vi "McPherson Setup for new pi.vi"(0 "Old GOTO":dbl format="%.2f", 2 "Old Begin":dbl format="%.2f", 4 "Old End":dbl format="%.2f", 7 "Duration":dbl format="%.2f", 9 "New Wavelength Unit":T1, 10 "Grating Density (g/mm)":T2=enum."1200" caption="Grating Density") -> (11 "Min Scan Time":dbl format="%.2f", 12 "StepperOutput":T3, 13 "Display":T4 {"Range"."Increment" format="%.2f"; "Range"."Maximum" format="%.2f"; "Range"."Minimum" format="%.2f"}, 14 "New GOTO":dbl format="%.2f", 16 "New Begin":dbl format="%.2f", 18 "New End":dbl format="%.2f", 19 "StepperGotoZ":i32)   [LabVIEW 2019]
uses:
  Globals and TypeDefs/Type Definitions.llb/McPherson Grating Density.ctl
  Globals and TypeDefs/Type Definitions.llb/Wavelength Unit.ctt
  File and save/X-Axis Converter.llb/X-Axis Converter.vi
panel:
  out "EndStep":i32
  out "BeginStep":i32
  out "Speed Output":i16
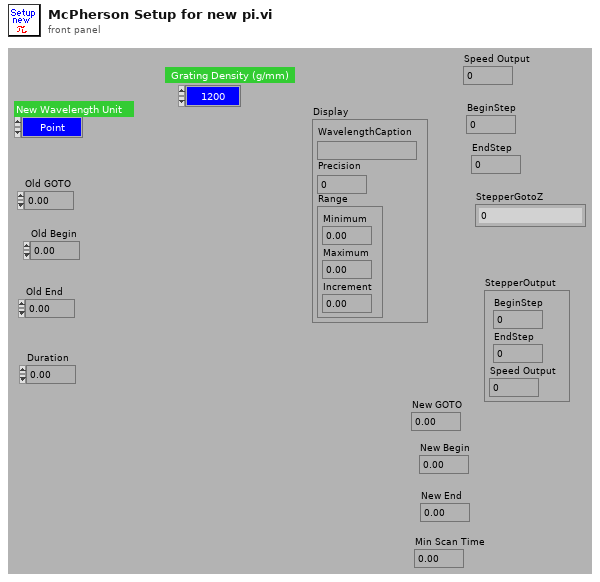
[diagram p1: front panel]
types:
  T1 = typedef "Wavelength Unit.ctt" = enum8{"Point", "nm", "eV", "meV", "cm_1"}
  T2 = typedef "McPherson Grating Density.ctl" = enum8{"150", "300", "600", "1200", "1800"}
  T3 = cluster{"BeginStep":i32, "EndStep":i32, "Speed Output":i16}
  T4 = cluster{"WavelengthCaption":string, "Precision":u8, "Range":cluster{"Minimum":dbl, "Maximum":dbl, "Increment":dbl}}
  T5 = cluster{"X-Axis Unit String":string, "Precision":i32, cluster{dbl, dbl, dbl}}
  T6 = cluster{"Stepper Position Output":i32, "Stepper Position Output":i32, i16}
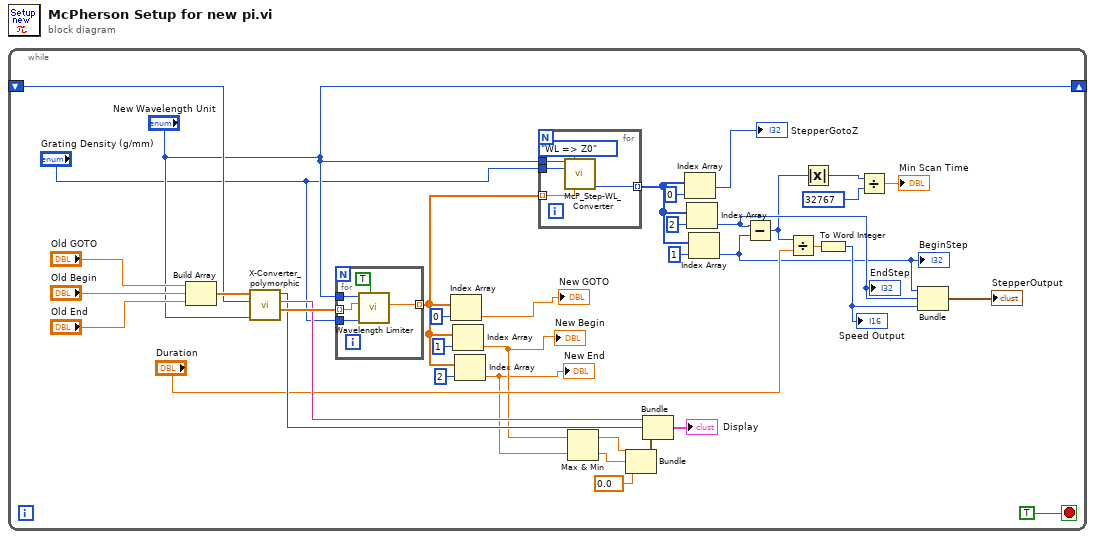
[diagram p0: block diagram]
diagram:
  n1 = while {
    shift-right: ["New Wavelength Unit"] -> _
    shift-left: _ -> [w12]
    stop <- TRUE stop-if-true
    n2 = Build Array("Old GOTO", "Old Begin", "Old End") -> (w15:dbl[])
    n3 = call-poly "X-Converter_polymorphic.vi"("X-Axis Unit"="New Wavelength Unit", "Old X-Axis Unit"=w12, "X-Axis input"=w15) -> ("X-Axis Output"=w36:dbl[], "X-Axis Unit String"=w24:string, "Precision"=w22:i32)  [unwired: 2 in, 1 out]
    n4 = for {
      tunnel: w36 -> [w48] mode=indexing
      tunnel: "New Wavelength Unit" -> [w47]
      tunnel: "Grating Density (g/mm)" -> [w46]
      tunnel: [w45] -> w32 mode=indexing
      n5 = call "Wavelength Limiter.vi"("Range Limiter(F) or WL limiter"=TRUE, "Current Grating Density"=w46, "Central WL Input"=w48, "X-Axis"=w47) -> ("Central WL output"=w45:dbl)  [unwired: 1 in, 3 out]
    }
    n6 = Index Array(array=w32, index=0 ("Index")) -> (element=→"New GOTO":dbl)
    n7 = Index Array(array=w32, index=1 ("Index")) -> (element=w8:dbl)
    "New Begin" <- w8
    n8 = Index Array(array=w32, index=2 ("Index")) -> (element=w7:dbl)
    "New End" <- w7
    n9 = for {
      tunnel: "New Wavelength Unit" -> [w43]
      tunnel: "Grating Density (g/mm)" -> [w42]
      tunnel: w32 -> [w41] mode=indexing
      tunnel: [w40] -> w28 mode=indexing
      n10 = call "McP_Step-WL_Converter.vi"("Wavelength Unit"=w43, "Option (Z0 <=> WL)"=enum16{"Z0 => WL", "WL => Z0", "Update WL only"}."WL => Z0", "Grating Density"=w42, "Wavelength Input"=w41) -> ("Stepper Position Output"=w40:i32)  [unwired: 4 in, 7 out]
    }
    n11 = Max & Min(x=w8, y=w7) -> (max(x,y)=w26:dbl, min(x,y)=w25:dbl)
    n12 = Bundle(w26, w25, 0.0) -> (w38:cluster{dbl, dbl, dbl})  [unwired: 1 in]
    n13 = Bundle("X-Axis Unit String"=w24, "Precision"=w22, w38) -> (→"Display":T5)  [unwired: 1 in]
    n14 = Index Array(array=w28, index=0 ("Index")) -> (element=→"StepperGotoZ":i32)
    n15 = Index Array(array=w28, index=2 ("Index")) -> (element=w6:i32)
    "EndStep" <- w6
    n16 = Index Array(array=w28, index=1 ("Index")) -> (element=w5:i32)
    "BeginStep" <- w5
    n17 = Subtract(x=w6, y=w5) -> (x-y=w4:i32)
    n18 = Divide(x=w4, y="Duration") -> (x/y=w27:dbl)
    n19 = Absolute Value(x=w4) -> (abs(x)=w3:i32)
    n20 = To Word Integer(number=w27) -> (16bit integer=w11:i16)
    "Speed Output" <- w11
    n21 = Divide(x=w3, y=32767 ("Velocity (Steps/s)")) -> (x/y=→"Min Scan Time":dbl)
    n22 = Bundle("Stepper Position Output"=w5, "Stepper Position Output"=w6, w11) -> (→"StepperOutput":T6)  [unwired: 1 in]
  }
